vi "read_attributes.vi"(8 "error in (no error)":errorcluster, 11 "BayesianRidge in":refnum<class "BayesianRidge.lvclass">) -> (0 "error out":errorcluster, 2 "attributes":T1, 3 "BayesianRidge out":refnum<class "BayesianRidge.lvclass">)   [LabVIEW 2020, in "BayesianRidge.lvclass"]
uses:
  BayesianRidge.lvclass
  Controls/bayesian_ridge_attributes.ctl
  BayesianRidge.lvclass/BayesianRidge.ctl
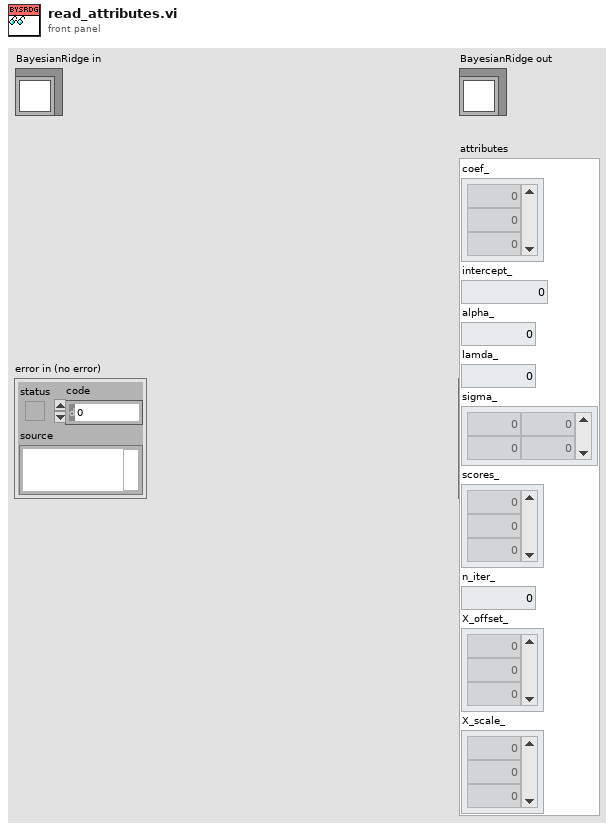
[diagram p1: front panel]
types:
  T1 = typedef "bayesian_ridge_attributes.ctl" = cluster{"coef_":dbl[], "intercept_":dbl, "alpha_":dbl, "lamda_":dbl, "sigma_":dbl[][], "scores_":dbl[], "n_iter_":dbl, "X_offset_":dbl[], "X_scale_":dbl[]}
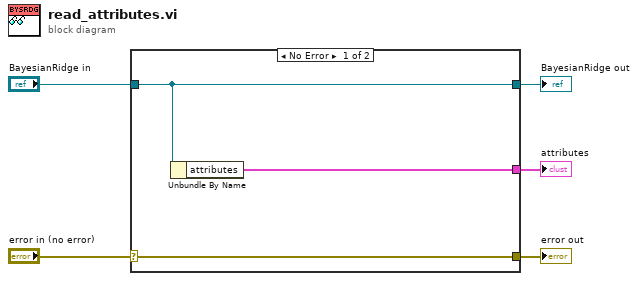
[diagram p0: block diagram]
diagram:
  n1 = case shown="No Error" "error in (no error)" {
    selector: "error in (no error)" -> [w8 w9]
    tunnel: [w8 w9] -> w4
    tunnel: [w7 w10] -> w2
    tunnel: "BayesianRidge in" -> [w7 w10]
    tunnel: [w6 _] -> w1
    frame No Error {
      n2 = Unbundle By Name(w7) -> ("attributes"=w6:T1)
    }
    frame Error {
    }
  }
  "error out" <- w4
  "BayesianRidge out" <- w2
  "attributes" <- w1
